vi "WS1050 16 DUT VSA-CV Sweep HD_Cycling_Ver1.4.vi"() -> ()   [LabVIEW 2012]
uses:
  WS_VCAP Driver 024/Source/WSVCAP Shell/Type Defs/WSVCAP SHL I2C DUT Mask Mode Enum.ctl
  <vilib>/Utility/file.llb/Read From Spreadsheet File (DBL).vi
  Type Def/Test Sequences.ctl
panel:
  out "VISA resource name out":refnum<visa-resource-name>="GPIB0::3::INSTR"
  out "date string":string="5/19/2014"
  out "PS1 Out":refnum<visa-resource-name>
  out "Ke2000 Out":refnum<visa-resource-name>="GPIB0::9::INSTR"
  in  "Tab Control":enum32{"Inst Control", "Data Output", "Graphs"}(tab)
  in  "Test Sequences":T1
  in  "Bank to HD":u16(ring) items=["All OFF", "All ON", "Bank_C1", "Bank_C2", "Bank_C3"]
  out "AD7747 Values":string[][](table)
  in  "Lot#":string="4NEMB"
  in  "Wafer#":string="20-EB"
  in  "File Name":string="HD_4NEMB_25_EB_65C_44V_100DC_BRD2_150916_1"
  in  "TMN DC\\CAP Data Log File Path":path=path "C:/WS1050 16 DUT Data"
  in  "SN":string[](array[string])=["1", "2", "3", "4", "5", "6", "7", "8", "9", "10", "11", "12", "13", "14", "15", "16"]
  in  "Test Program":string="WS1050 16 DUT VSA_CV Sweep HD_Cycling Ver1.4"
  out "Current Date":string="8/28/2014"
  out "Current Time":string="0950"
  in  "Start Date":string="4/24/2014"
  in  "Start Time":string="1542"
  in  "Comment":string="CV Sweep"
  in  "OK Button":bool
  in  "Calibration":bool
  in  "Control Setting":bool
  in  "CP Setting":i32(ring) items=["CP OFF", "CP ON", "CP 35V", "CP 40V", "CP 44V", "CP 50V", "DVA OFF", "DVA ON", "Reg1 ON", "Reg1 OFF", "Reg2 ON", "Reg2 OFF", "Reg3 ON", "Reg3 OFF"]
  in  "VDD(V)":dbl=3.3 format="%.3g"
  in  "Meas Clock Rate (Hz)":dbl=1000000.0 caption="Meas Speed" format="%.1p Hz"
  out "AR  Measurent(Hz)":dbl
  in  "PS1 Source":refnum<visa-resource-name>="GPIB0::5::INSTR"
  in  "Ke2000":refnum<visa-resource-name>="GPIB0::9::INSTR"
  out "Simulate FPGA":bool
  out "Online":bool
  in  "Ke2400":refnum<visa-resource-name>="GPIB0::3::INSTR"
  in  "Initialize AD7747":bool
  in  "DUT Mask Mode":T2=enum."All"
  in  "RFFE Slave Address":u8=7 caption="Slave Address" format="0x%02x"
  out "Activity Log":string="05/19/2014 -- 12:24:35.853::WSVCAP::APP::Application Started\n05/19/2014 -- 12:24:37.606::WSVCAP::WSVCAP SHL::WR I2C-REG:0x0A;MASK:0xFFFFFFFFFFFF;C1 DATA:22:22:22:22:22:22:22:22:22:22:22:22:22:22:22:22;C2 DATA:22:22:22:22:22:22:22:22:22:22:22:22:22:22:22:22;C3 DATA:22:22:22:22:22:22:22:22:22:22:22:22:22:22:22:22\r\n05/19/2014 -- 12:24:37.773::WSVCAP::WSVCAP SHL::WR I2C-ST:0,0,4,1\r\n05/19/2014 -- 12:24:37.903::WSVCAP::WSVCAP SHL::RD I2C-BYTES:4;ADD:0x00;MASK:0xFFFFFFFFFFFF\r\n05/19/2014 -- 12:24:38.045::WSVCAP::WSVCAP SHL::RD I2C:C1 DATA:2:2:2:2:2:2:2:2:2:2:2:2:2:2:2:2|A7:A9:AA:82:82:7F:82:81:82:81:83:82:81:82:82:81|46:36:BB:88:44:A3:E9:2B:32:20:ED:25:BB:3D:68:B|2C:6A:EB:A7:22:56:FE:CC:36:82:D7:B0:3B:48:F9:CC;C2 DATA:2:2:2:2:2:2:2:2:2:2:2:2:2:2:2:2|94:94:94:80:80:80:80:80:81:7E:7E:81:80:7E:80:80|47:33:15:82:62:B:E8:1C:D7:C3:7D:41:7C:B7:4C:2A|C4:B4:AE:8:1E:D1:4E:37:11:C0:6F:63:42:9D:63:B5;C3 DATA:2:2:2:2:2:2:2:2:2:2:2:2:2:2:2:2|95:95:95:81:81:7E:81:80:84:7D:80:83:81:7E:7F:80|AB:C4:14:B5:7B:52:DF:C9:79:5D:5F:30:99:31:1E:F4|6E:5C:F7:A8:C3:EB:7B:EF:33:92:89:77:4D:67:75:DD;STATUS:0:0:4:0\r\n05/19/2014 -- 12:24:38.046::WSVCAP::WSVCAP SHL::WR I2C-REG:0x0A;MASK:0xFFFFFFFFFFFF;C1 DATA:22:22:22:22:22:22:22:22:22:22:22:22:22:22:22:22;C2 DATA:22:22:22:22:22:22:22:22:22:22:22:22:22:22:22:22;C3 DATA:22:22:22:22:22:22:22:22:22:22:22:22:22:22:22:22\r\n05/19/2014 -- 12:24:38.089::WSVCAP::WSVCAP SHL::WR I2C-ST:0,0,4,1\r\n05/19/2014 -- 12:24:38.219::WSVCAP::WSVCAP SHL::RD I2C-BYTES:4;ADD:0x00;MASK:0xFFFFFFFFFFFF\r\n05/19/2014 -- 12:24:38.362::WSVCAP::WSVCAP SHL::RD I2C:C1 DATA:2:2:2:2:2:2:2:2:2:2:2:2:2:2:2:2|A7:AB:AA:82:82:82:83:83:82:82:82:82:7F:82:82:81|4B:32:96:83:3E:61:43:17:25:62:AB:4D:A2:40:2E:5|3C:76:2B:B4:EE:E4:A9:1A:AA:A:26:C7:21:2E:87:5B;C2 DATA:2:2:2:2:2:2:2:2:2:2:2:2:2:2:2:2|94:94:94:80:80:80:80:80:80:7F:80:81:80:80:7F:80|4A:32:19:7D:19:6C:79:46:61:7F:4B:B8:A5:30:F3:14|B4:70:A:8C:9C:DC:43:FA:1E:A:C6:21:A:A9:13:F3;C3 DATA:2:2:2:2:2:2:2:2:2:2:2:2:2:2:2:2|95:97:94:81:80:81:82:81:80:7E:81:84:7F:81:80:80|B2:32:D0:A7:9E:4C:AB:D4:EE:D9:F0:82:B7:91:7:FF|C1:91:B6:3D:D8:E:1B:4F:9F:6A:F1:6C:E7:3F:7:BA;STATUS:0:0:4:0\r\n05/19/2014 -- 12:24:38.364::WSVCAP::WSVCAP SHL::WR I2C-REG:0x0A;MASK:0xFFFFFFFFFFFF;C1 DATA:22:22:22:22:22:22:22:22:22:22:22:22:22:22:22:22;C2 DATA:22:22:22:22:22:22:22:22:22:22:22:22:22:22:22:22;C3 DATA:22:22:22:22:22:22:22:22:22:22:22:22:22:22:22:22\r\n05/19/2014 -- 12:24:38.406::WSVCAP::WSVCAP SHL::WR I2C-ST:0,0,4,1\r\n05/19/2014 -- 12:24:38.536::WSVCAP::WSVCAP SHL::RD I2C-BYTES:4;ADD:0x00;MASK:0xFFFFFFFFFFFF\r\n05/19/2014 -- 12:24:38.678::WSVCAP::WSVCAP SHL::RD I2C:C1 DATA:2:2:2:2:2:2:2:2:2:2:2:2:2:2:2:2|A7:A9:AB:82:82:81:82:82:82:82:82:82:82:82:82:81|46:71:4C:87:43:3D:7F:FC:25:4F:8E:54:97:3E:60:8C|AA:F4:1F:B5:CE:43:1F:36:9:87:9C:78:86:5:B6:8E;C2 DATA:2:2:2:2:2:2:2:2:2:2:2:2:2:2:2:2|94:94:94:80:7F:7F:80:80:80:80:80:81:80:80:80:80|49:36:18:7D:6E:C5:E4:3C:81:2E:41:D3:75:71:E3:72|E8:D3:E6:D1:E0:48:AE:D4:54:D:E8:8E:B4:41:68:4;C3 DATA:2:2:2:2:2:2:2:2:2:2:2:2:2:2:2:2|95:95:95:81:7F:7F:81:81:81:81:81:84:81:81:82:81|B3:F5:90:AB:82:69:7B:93:D0:77:E8:D5:E8:8C:84:E8|B9:AC:EE:2B:B6:71:8F:4A:74:31:56:BB:8A:B7:A0:C8;STATUS:0:0:4:0\r\n05/19/2014 -- 12:24:38.681::WSVCAP::WSVCAP SHL::WR I2C-REG:0x0A;MASK:0xFFFFFFFFFFFF;C1 DATA:22:22:22:22:22:22:22:22:22:22:22:22:22:22:22:22;C2 DATA:22:22:22:22:22:22:22:22:22:22:22:22:22:22:22:22;C3 DATA:22:22:22:22:22:22:22:22:22:22:22:22:22:22:22:22\r\n05/19/2014 -- 12:24:38.723::WSVCAP::WSVCAP SHL::WR I2C-ST:0,0,4,1\r\n05/19/2014 -- 12:24:38.854::WSVCAP::WSVCAP SHL::RD I2C-BYTES:4;ADD:0x00;MASK:0xFFFFFFFFFFFF\r\n05/19/2014 -- 12:24:38.996::WSVCAP::WSVCAP SHL::RD I2C:C1 DATA:2:2:2:2:2:2:2:2:2:2:2:2:2:2:2:2|A7:A9:AA:82:82:7F:83:81:82:81:84:82:7F:82:7F:82|43:FB:E:7F:3C:AD:35:35:26:A2:6C:21:4B:3D:8:6|63:9A:E1:F3:95:32:91:42:90:3C:78:1F:5C:D7:5F:D8;C2 DATA:2:2:2:2:2:2:2:2:2:2:2:2:2:2:2:2|94:94:94:80:80:80:80:80:81:80:7E:81:80:7E:7F:80|48:36:18:7F:5E:3D:69:83:DE:AE:A1:9E:31:AE:BB:96|15:A0:44:17:13:FD:CC:C8:6D:B2:EF:A7:C:C7:3B:F;C3 DATA:2:2:2:2:2:2:2:2:2:2:2:2:2:2:2:2|95:96:94:81:81:7E:82:80:84:80:80:84:7F:7E:7D:82|AD:3B:6D:A9:7C:57:9D:F5:7A:96:23:5C:36:2D:ED:5A|CD:46:DB:3B:C7:BD:70:60:33:B8:B:F7:63:A:51:4D;STATUS:0:0:4:0\r\n05/19/2014 -- 12:24:38.998::WSVCAP::WSVCAP SHL::WR I2C-REG:0x0A;MASK:0xFFFFFFFFFFFF;C1 DATA:22:22:22:22:22:22:22:22:22:22:22:22:22:22:22:22;C2 DATA:22:22:22:22:22:22:22:22:22:22:22:22:22:22:22:22;C3 DATA:22:22:22:22:22:22:22:22:22:22:22:22:22:22:22:22\r\n05/19/2014 -- 12:24:39.040::WSVCAP::WSVCAP SHL::WR I2C-ST:0,0,4,1\r\n05/19/2014 -- 12:24:39.170::WSVCAP::WSVCAP SHL::RD I2C-BYTES:4;ADD:0x00;MASK:0xFFFFFFFFFFFF\r\n05/19/2014 -- 12:24:39.311::WSVCAP::WSVCAP SHL::RD I2C:C1 DATA:2:2:2:2:2:2:2:2:2:2:2:2:2:2:2:2|A7:AA:AB:82:82:81:82:81:82:81:82:82:82:82:7F:82|44:F1:90:87:45:44:C8:2C:2C:F1:FC:1B:94:3B:3C:75|4A:49:95:19:99:73:64:3:23:24:F3:A2:5E:7F:C4:B6;C2 DATA:2:2:2:2:2:2:2:2:2:2:2:2:2:2:2:2|94:94:94:80:80:80:80:7F:80:80:7E:80:80:7E:7F:80|4C:36:17:7D:A8:9F:DE:C7:53:6D:8A:F4:41:A5:C6:E0|90:2E:24:C:D9:22:E4:76:3B:40:1D:53:33:B1:3E:4D;C3 DATA:2:2:2:2:2:2:2:2:2:2:2:2:2:2:2:2|95:97:95:81:81:7F:81:80:80:81:7F:82:81:7E:7D:82|AE:2B:A7:AB:CC:CD:A4:38:FD:17:80:F2:92:2D:45:C4|76:E5:D:B9:AD:B5:BA:8D:28:32:9E:42:B7:20:4A:D9;STATUS:0:0:4:0\r\n05/19/2014 -- 12:24:39.313::WSVCAP::WSVCAP SHL::WR I2C-REG:0x0A;MASK:0xFFFFFFFFFFFF;C1 DATA:22:22:22:22:22:22:22:22:22:22:22:22:22:22:22:22;C2 DATA:22:22:22:22:22:22:22:22:22:22:22:22:22:22:22:22;C3 DATA:22:22:22:22:22:22:22:22:22:22:22:22:22:22:22:22\r\n05/19/2014 -- 12:24:39.355::WSVCAP::WSVCAP SHL::WR I2C-ST:0,0,4,1\r\n05/19/2014 -- 12:24:39.486::WSVCAP::WSVCAP SHL::RD I2C-BYTES:4;ADD:0x00;MASK:0xFFFFFFFFFFFF\r\n05/19/2014 -- 12:24:39.628::WSVCAP::WSVCAP SHL::RD I2C:C1 DATA:2:2:2:2:2:2:2:2:2:2:2:2:2:2:2:2|A7:A9:AA:82:82:82:83:82:82:82:82:82:7F:82:7F:82|47:18:E4:87:3E:E7:6:65:25:92:37:38:A8:3E:89:85|7C:A7:7:2B:A3:7A:EC:EF:89:ED:F4:D3:D8:BC:3A:F5;C2 DATA:2:2:2:2:2:2:2:2:2:2:2:2:2:2:2:2|94:94:94:80:7F:80:80:7F:81:80:7E:80:80:80:81:80|49:37:17:80:76:25:6A:F8:DF:55:97:4D:B8:5B:2B:B1|13:E3:9A:3E:1A:2D:4F:B6:DB:E9:61:FA:8B:D6:9:CC;C3 DATA:2:2:2:2:2:2:2:2:2:2:2:2:2:2:2:2|95:95:95:81:7F:80:82:81:84:80:7F:81:80:81:7F:82|AF:93:3B:AF:5B:11:82:E4:7E:C3:2D:72:9:96:D9:A|DB:96:F2:10:5F:64:9A:C6:98:12:27:7D:10:D3:20:D9;STATUS:0:0:4:0\r\n05/19/2014 -- 12:24:40.132::WSVCAP::WSVCAP SHL::CLOSE\r\n"
  in  "C1 Cap DAC":u8=128 caption="B Data In" format="0x%02x"
  in  "C2 Cap DAC":u8=128 caption="B Data In" format="0x%02x"
  in  "C3 Cap DAC":u8=128 caption="B Data In" format="0x%02x"
  out "IDD Brd(uA)":string
  in  "VSA_IDD(A)":dbl=0.1
  in  "Stress Voltage(V)":dbl
  in  "Reset PS":bool
  in  "CP Freq":u16(ring)=3 items=["000", "001", "010", "011", "100", "101", "110", "111"]
  in  "HD/Cycling":bool
  in  "Cyc Clock Rate (Hz)":dbl=5000000.0 caption="Cycle Speed" format="%.1p Hz"
  in  "CP to HD/Cycle":i32(ring)=4 items=["CP HDC 35V", "CP HDC 40.25V", "CP HDC 27.5V", "CP HDC 30.5V", "CP HDC 44V", "CP HDC 50V"]
  in  "Bank to Cycle":u16(ring)=1 items=["Cycle All", "Cycle F12+S1", "Cycle All - F12"]
  in  "Duty Cycle %":enum16{"25", "33", "50", "75"}(ring)=enum."50"
  out "STATUS":string="Idle...."
  in  "stop":bool
  out "C1 Min_T0":string[](array[string])
  out "CAP_Value(pF)":string[][](array[string])
  out "C3 Min_T0":string[](array[string])
  out "C2 Min_T0":string[](array[string])
  in  "Abort":bool
  out "error out 2":errorcluster
  in  "Set Stress to\nComplete(Cyc/Min)":u64=8100
  out "Verify Test Condition":string[](array[string])
  out "CMin+VCAP":string[][](table)
  out "Verify Drivers to Stress":string[](array[string])
  out "Cycle Count":u64 min=1 max=4 step=1
  out "Stress \nCompleted(Min)":u64
  out "Previous Time":string="12:20:26 PM"
  out "Delta CAP_T0(pF)":dbl[][](array[numeric])
  out "Delta CAP_Tc(pF)":dbl[][](array[numeric])
  in  "error in (no error)":errorcluster
  out "error out":errorcluster
  out "CP_IDD(uA)":string
  # "Company:  WiSpry Inc 20 Fairbanks \nSte 198 Irvine CA 92618\n\nAuthor:  Andy V Tran\nCreated:  01/07/2016\nLabVIEW 2012 Pro\nTP:  WS1050 16 DUT VSA_CV Sweep HD_Cycling Ver1.3\nFPGA Version: WS_VCAP Driver 024"
  # "Note:  Ver1.0 is a original version.\n\n1.  Two look up tables, \n      a.  1st is for Stress\n      b.  2nd is for Voltage sweep\n\nVer1.1\n\n1.  No Voltage to CAP Head for initial read point\n\nVer1.2\n\n1.  Add CP Freq\n\nVer1.3\n\n1.  Add Cycling Stress\n\nSet up and Test Sequences:\n\n1.  Calibration with Empty Sockets\n2.  Load Parts\n3.  Set condition to stress (CP Voltage, Drivers to Stress, CP to stress...)\n4.  Set Date/Time to start stressing\n5.  Set TTF to stop stressing (default = 135 hrs)"
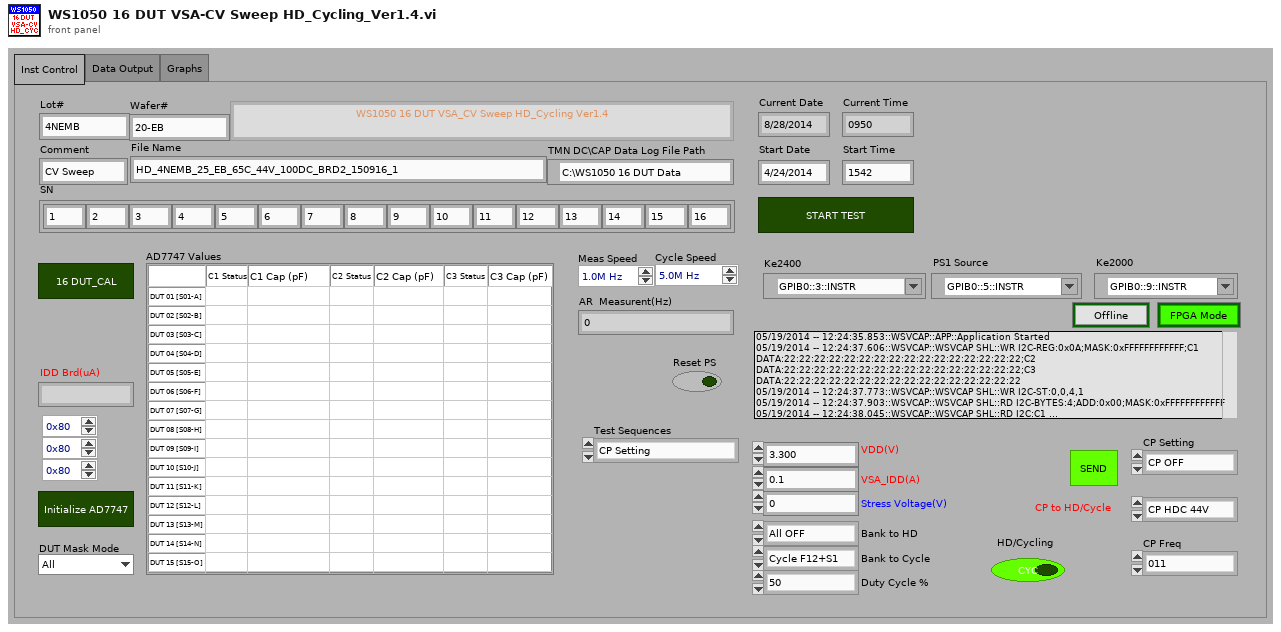
[diagram p1: front panel]
types:
  T1 = typedef "Test Sequences.ctl" = enum16{"CP Setting", "Stress", "Meas_IDD", "Meas_Cap", "Save Data", "Plot", "Idle..."}
  T2 = typedef "WSVCAP SHL I2C DUT Mask Mode Enum.ctl" = enum16{"Custom", "C1", "C2", "C3", "All"}
  T3 = typedef "WSVCAP SHL Core System Cluster.ctl" = cluster{"Settings":T4, "FPGA Resource":tag, "Online":bool, "I2C Wait Ticks":u32, "SPI Wait Ticks":u32, "RFFE Wait Ticks":u32}
  T4 = typedef "WSVCAP SHL I2C Settings Cluster.ctl" = cluster{"FPGA Resource Name":string, "I2C Slave Address":u8, "I2C Clock Rate (Hz)":dbl, "SPI Clock Rate (Hz)":dbl, "RFFE Slave Address":u8, "RFFE Clock Rate (Hz)":dbl, "Simulate FPGA":bool, "C1 Cap DAC Default":u8, "C2 Cap DAC Default":u8, "C3 Cap DAC Default":u8}
  T5 = enum16{"Idle...", "Voltage 1", "Voltage 2", "Voltage 3"}[]
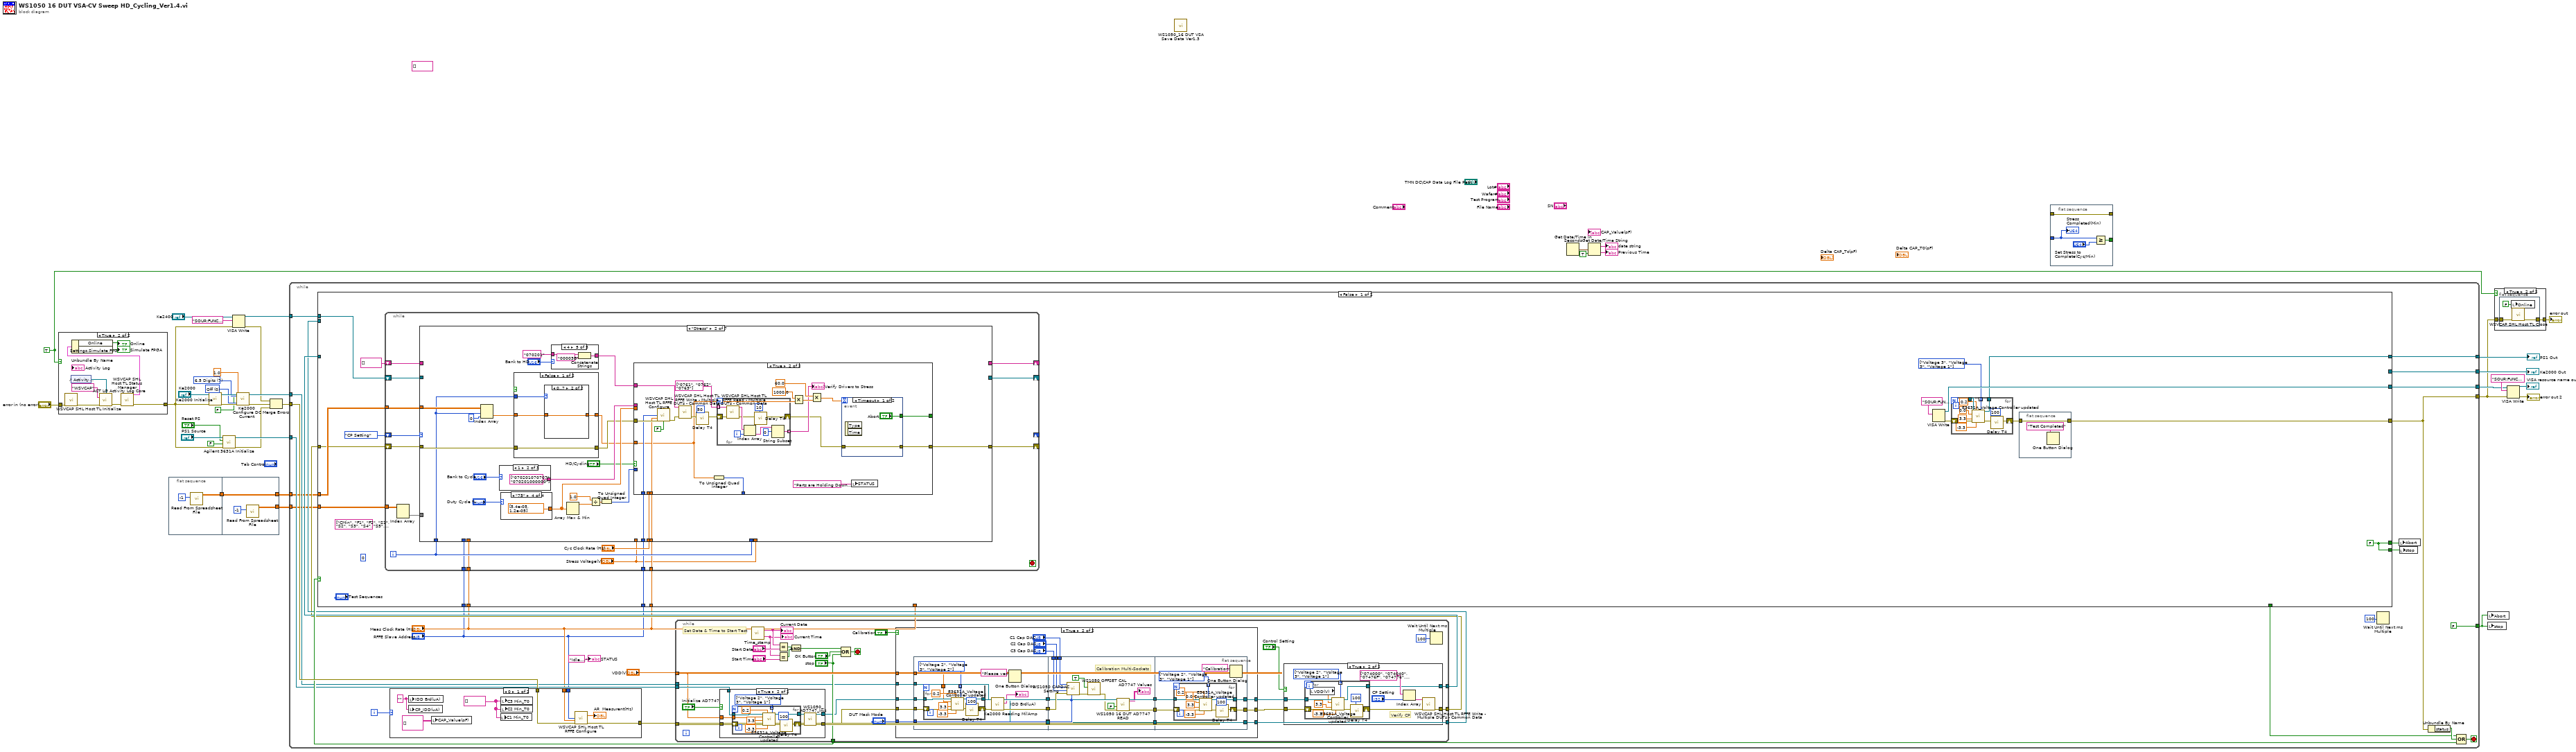
[diagram p0: block diagram]
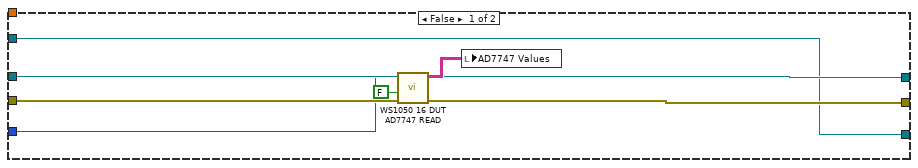
[diagram p7: hidden frame]
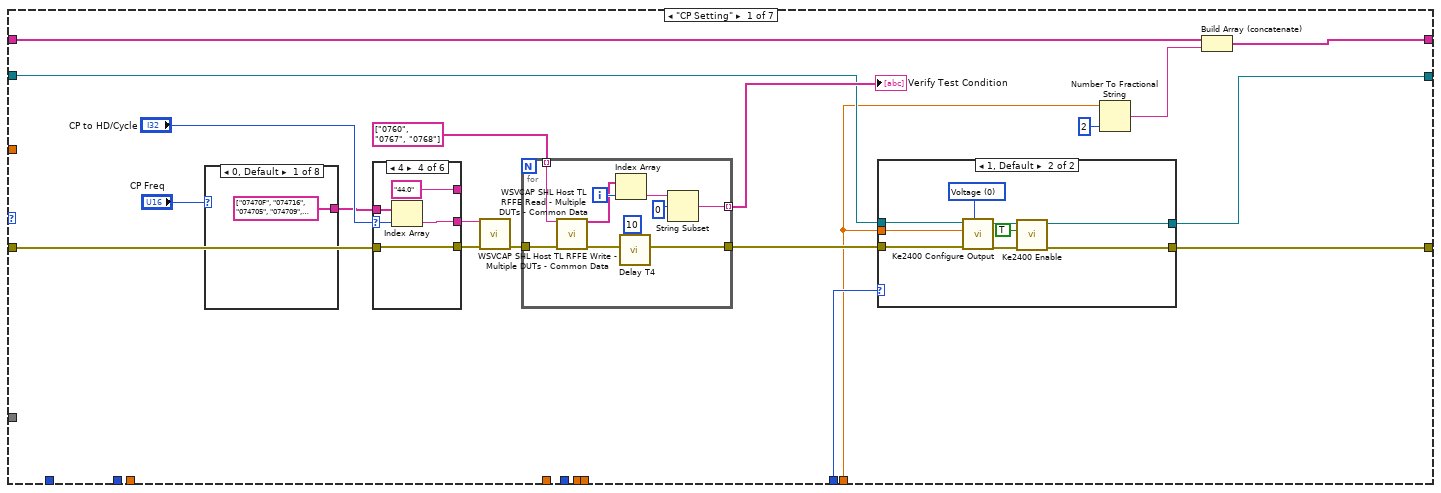
[diagram p8: hidden frame]
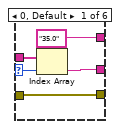
[diagram p10: hidden frame]
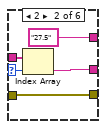
[diagram p11: hidden frame]
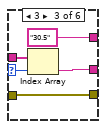
[diagram p12: hidden frame]
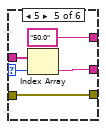
[diagram p13: hidden frame]
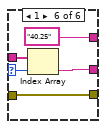
[diagram p14: hidden frame]
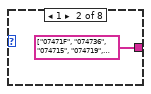
[diagram p15: hidden frame]
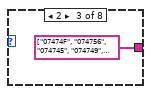
[diagram p16: hidden frame]
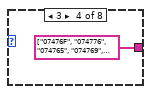
[diagram p17: hidden frame]
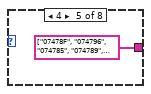
[diagram p18: hidden frame]
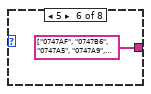
[diagram p19: hidden frame]
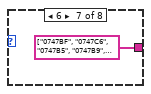
[diagram p20: hidden frame]
diagram:
  (unwired) string[] []
  w30 = TRUE
  w36 = u16 0 items=["Off", "Moving Filter", "Repeating Filter"] ("Digital Filter (0: Off)")
  w37 = u16 7 items=["3.5 Digits"=4, "4.5 Digits"=5, "5.5 Digits"=6, "6.5 Digits"=7] ("Resolution (7: 6.5 digits)")
  n1 = case shown="True" w30 {
    tunnel: "error in (no error)" -> [w44 w45]
    tunnel: [w44 w52] -> w19
    frame False {
    }
    frame True {
      n2 = call "WSVCAP SHL Host TL Initialize.vi"("error in"=w45) -> ("error out"=w46:errorcluster)  [unwired: 13 in, 1 out]
      n3 = control-ref of="Activity Log"() -> (w48:refnum<vi>)
      n4 = call "ACT LG Activity Log Core.vi"("Display Ref"=w48, "Source"="WSVCAP", "Error In (no error)"=w46) -> ("Error Out"=w47:errorcluster)  [unwired: 11 in, 1 out]
      n5 = call "WSVCAP SHL Host TL Status Manager.vi"("error in"=w47) -> ("System Out"=w53:T3, "error out"=w52:errorcluster)  [unwired: 13 in]
      n6 = Unbundle By Name(w53) -> ("Online"=→"Online":bool, "Settings.Simulate FPGA"=→"Simulate FPGA":bool)
    }
  }
  n7 = flat-sequence {
    tunnel: [w55] -> w14
    tunnel: w14 -> [w58]
    tunnel: [w58] -> w13
    tunnel: [w57] -> w12
    frame #0 {
      n8 = call-poly <vilib>:"Read From Spreadsheet File.vi"("number of rows (all:-1)"=-1) -> ("all rows"=w55:dbl[][])  [unwired: 6 in, 4 out]
    }
    frame #1 {
      n9 = call-poly <vilib>:"Read From Spreadsheet File.vi"("number of rows (all:-1)"=-1) -> ("all rows"=w57:dbl[][])  [unwired: 6 in, 4 out]
    }
  }
  n10 = call "Ke2000 Initialize.vi"("error in (no error)"=w19, "VISA resource name"="Ke2000") -> ("error out"=w38:errorcluster, "VISA resource name out"=w39:refnum<visa-resource-name>)  [unwired: 8 in]
  n11 = call "Agilent 3631A Initialize.vi"("error in (no error)"=w19, "Default"=FALSE ("Reset? (T: Yes)"), "Reset"="Reset PS", "VISA resource name"="PS1 Source") -> ("error out"=w18:errorcluster, "VISA resource name out"=w42:refnum<visa-resource-name>)  [unwired: 6 in]
  n12 = VISA Write(VISA resource name="Ke2400", write buffer="SOUR:FUNC VOLT;VOLT:MODE FIX;RANG 100;LEV 0.0;:SENS:FUNC \"CURR\";CURR:PROT 60E-3;RANG 100E-3;:OUTP ON", error in (no error)=w19) -> (VISA resource name out=w27:refnum<visa-resource-name>, error out=w22:errorcluster)  [unwired: 1 out]
  n13 = call "Ke2000 Configure DC Current.vi"("Resolution (7: 6.5 digits)"=w37, "Digital Filter (0: Off)"=w36, "Auto Range? (T: Auto)"=FALSE, "error in"=w38, "Custom Range (0 A)"=1.0, "VISA resource name"=w39) -> ("error out"=w20:errorcluster, "VISA resource name out"=w34:refnum<visa-resource-name>)  [unwired: 4 in]
  n14 = Merge Errors(w22, w20, w18) -> (w28:errorcluster)
  n15 = while {
    tunnel: w28 -> [w79]
    tunnel: [w69] -> w24
    tunnel: w42 -> [w73]
    tunnel: w34 -> [w74]
    tunnel: [w82] -> w33
    tunnel: [w81] -> w32
    tunnel: w27 -> [w78]
    tunnel: [w77] -> w25
    tunnel: [FALSE] -> w17
    tunnel: w13 -> [w65]
    tunnel: w12 -> [w64]
    i -> [w80]
    stop <- w83 stop-if-true
    n16 = case shown="0" w80 {
      tunnel: w79 -> [w93 w94]
      tunnel: [w92 w94] -> w75
      tunnel: "RFFE Slave Address" -> [w90 _]
      tunnel: "Meas Clock Rate (Hz)" -> [w86 _]
      frame 0 {
        w89 = string[] []
        w87 = "" ("uA")
        n17 = local write "IDD Brd(uA)"(w87) -> ()
        n18 = local write "CP_IDD(uA)"(w87) -> ()
        n19 = local write "CAP_Value(pF)"(string[][] []) -> ()
        n20 = local write "C1 Min_T0"(w89) -> ()
        n21 = local write "C3 Min_T0"(w89) -> ()
        n22 = local write "C2 Min_T0"(w89) -> ()
        n23 = call "WSVCAP SHL Host TL RFFE Configure.vi"("RFFE Slave Address"=w90, "Clock Rate (Hz)"=w86, "error in"=w93) -> ("Actual Rate (Hz)"=→"AR  Measurent(Hz)":dbl, "error out"=w92:errorcluster)  [unwired: 11 in]
      }
      frame 1, Default {
      }
    }
    n24 = while {
      tunnel: ["stop"] -> w76
      tunnel: w75 -> [w106]
      tunnel: [w98] -> w70
      tunnel: w73 -> [w104]
      tunnel: w74 -> [w100]
      tunnel: [w101] -> w72
      tunnel: [w99] -> w71
      tunnel: "VDD(V)" -> [w96]
      stop <- w113 stop-if-true
      # "Set Date & Time to Start Test"
      n25 = case shown="True" "Initialize AD7747" {
        tunnel: w106 -> [w122 w128]
        tunnel: [w122 w124] -> w105
        tunnel: w104 -> [w121 w126]
        tunnel: [w121 w125] -> w103
        tunnel: w96 -> [_ w123]
        frame False {
        }
        frame True {
          w129 = T5 [enum."Voltage 2", enum."Voltage 3", enum."Voltage 1"] items=["Idle...", "Voltage 1", "Voltage 2", "Voltage 3"]
          n26 = for {
            tunnel: w126 -> [w139]
            tunnel: w129 -> [w137] mode=indexing
            tunnel: [w136] -> w125
            shift-right: [w133] -> w127
            shift-left: w128 -> [w140]
            tunnel: w123 -> [w131]
            n27 = call "E3631A_Voltage Controller updated.vi"("VISA resource name"=w139, "I_VDD(A)"=0.2, "Channel Controller"=w137, "Voltage 1"=w131, "Voltage 2"=3.3, "error in (no error)"=w140, "Voltage 3"=-3.3) -> ("VISA resource name out"=w136:refnum<visa-resource-name>, "error out"=w132:errorcluster)  [unwired: 7 in]
            n28 = call "Delay T4.vi"("milliseconds to wait"=u32 100, "error in (no error)"=w132) -> ("error out"=w133:errorcluster)  [unwired: 9 in]
          }
          n29 = call "WS1050_AD7747_Init.vi"("error in"=w127) -> ("error out"=w124:errorcluster)  [unwired: 10 in]
        }
      }
      n30 = call "Time_stamp.vi"() -> ("date/time string"=w118:string, "date string"=w120:string)  [unwired: 2 in]
      "Current Date" <- w120
      "Current Time" <- w118
      n31 = Equal?(x=w120, y="Start Date") -> (x = y?=w116:bool)
      n32 = Equal?(x=w118, y="Start Time") -> (x = y?=w115:bool)
      n33 = And(x=w116, y=w115) -> (x .and. y?=w112:bool)
      n34 = Compound Arithmetic op=OR(w112, "OK Button", "stop") -> (w113:bool)
      n35 = case shown="True" "Calibration" {
        tunnel: w105 -> [w167 w186]
        tunnel: [w166 w183] -> w97
        tunnel: w103 -> [w165 w182]
        tunnel: "DUT Mask Mode" -> [w164 w178]
        tunnel: [w165 w177] -> w102
        tunnel: w100 -> [w163 w173]
        tunnel: [w163 w170] -> w99
        tunnel: w96 -> [_ w169]
        frame False {
          n36 = call "WS1050 16 DUT AD7747 READ.vi"("error in"=w167, "Log (T)"=FALSE, "DUT Mask Mode (All)"=w164) -> ("error out"=w166:errorcluster, "AD7747 Values"=w168:string[][])  [unwired: 7 in]
          n37 = local write "AD7747 Values"(w168) -> ()
        }
        frame True {
          n38 = flat-sequence {
            tunnel: w186 -> [w196]
            tunnel: [w191] -> w185
            tunnel: w182 -> [w195]
            tunnel: [w194] -> w181
            tunnel: w178 -> [w193]
            tunnel: [w193] -> w179
            tunnel: w173 -> [w189]
            tunnel: [w188] -> w172
            tunnel: w169 -> [w187]
            tunnel: w185 -> [w222]
            tunnel: [w221] -> w184
            tunnel: w181 -> [w220]
            tunnel: [w220] -> w180
            tunnel: w179 -> [w219]
            tunnel: "C1 Cap DAC" -> [w215]
            tunnel: "C2 Cap DAC" -> [w214]
            tunnel: "C3 Cap DAC" -> [w213]
            tunnel: w172 -> [w212]
            tunnel: [w212] -> w171
            tunnel: w184 -> [w225]
            tunnel: [w228] -> w183
            tunnel: w180 -> [w227]
            tunnel: [w224] -> w177
            tunnel: w171 -> [w223]
            tunnel: [w223] -> w170
            frame #0 {
              w197 = T5 [enum."Voltage 2", enum."Voltage 3", enum."Voltage 2"] items=["Idle...", "Voltage 1", "Voltage 2", "Voltage 3"]
              n39 = for {
                tunnel: w195 -> [w208]
                tunnel: w197 -> [w205] mode=indexing
                tunnel: [w204] -> w194
                shift-right: [w202] -> w190
                shift-left: w196 -> [w209]
                tunnel: w187 -> [w199]
                n40 = call "E3631A_Voltage Controller updated.vi"("VISA resource name"=w208, "I_VDD(A)"=0.2, "Channel Controller"=w205, "Voltage 1"=w199, "Voltage 2"=3.3, "error in (no error)"=w209, "Voltage 3"=-3.3) -> ("VISA resource name out"=w204:refnum<visa-resource-name>, "error out"=w201:errorcluster)  [unwired: 7 in]
                n41 = call "Delay T4.vi"("milliseconds to wait"=u32 100, "error in (no error)"=w201) -> ("error out"=w202:errorcluster)  [unwired: 9 in]
              }
              n42 = call "Ke2000 Reading MilAmp.vi"("error in (no error)"=w190, "VISA resource name"=w189) -> ("error out"=w191:errorcluster, "uA"=→"IDD Brd(uA)":string, "VISA resource name out"=w188:refnum<visa-resource-name>)  [unwired: 7 in]
              n43 = One Button Dialog(message="Please verify all sockets should be empty...") -> ()  [unwired: 1 in, 1 out]
            }
            frame #1 {
              # "Calibration Multi-Sockets"
              n44 = call "WS1050 CAPDAC Setting.vi"("DUT Mask Mode (All)"=w219, "error in"=w222, "C3 Cap DAC"=w213, "C2 Cap DAC"=w214, "C1 Cap DAC"=w215) -> ("error out"=w217:errorcluster)  [unwired: 5 in, 1 out]
              n45 = call "WS1050 OFFSET CAL.vi"("error in"=w217, "OFFSET CAL"=TRUE ("Read?")) -> ("error out"=w216:errorcluster)  [unwired: 8 in, 1 out]
              n46 = call "WS1050 16 DUT AD7747 READ.vi"("error in"=w216, "Log (T)"=FALSE, "DUT Mask Mode (All)"=w219) -> ("error out"=w221:errorcluster, "AD7747 Values"=→"AD7747 Values":string[][])  [unwired: 7 in]
            }
            frame #2 {
              w226 = T5 [enum."Voltage 2", enum."Voltage 3", enum."Voltage 1"] items=["Idle...", "Voltage 1", "Voltage 2", "Voltage 3"]
              n47 = for {
                tunnel: w227 -> [w240]
                tunnel: w226 -> [w236] mode=indexing
                tunnel: [w235] -> w224
                shift-right: [w231] -> w228
                shift-left: w225 -> [w237]
                n48 = call "E3631A_Voltage Controller updated.vi"("VISA resource name"=w240, "I_VDD(A)"=0.2, "Channel Controller"=w236, "Voltage 1"=0.0, "Voltage 2"=3.3, "error in (no error)"=w237, "Voltage 3"=-3.3) -> ("VISA resource name out"=w235:refnum<visa-resource-name>, "error out"=w230:errorcluster)  [unwired: 7 in]
                n49 = call "Delay T4.vi"("milliseconds to wait"=u32 100, "error in (no error)"=w230) -> ("error out"=w231:errorcluster)  [unwired: 9 in]
              }
              n50 = One Button Dialog(message="Calibration Completed....") -> ()  [unwired: 1 in, 1 out]
            }
          }
        }
      }
      n51 = case shown="True" "Control Setting" {
        tunnel: [w141 w144] -> w98
        tunnel: w102 -> [w142 w147]
        tunnel: [w142 w145] -> w101
        tunnel: w97 -> [w141 w143]
        frame False {
        }
        frame True {
          w148 = T5 [enum."Voltage 2", enum."Voltage 3", enum."Voltage 1"] items=["Idle...", "Voltage 1", "Voltage 2", "Voltage 3"]
          # "Verify CP"
          n52 = for {
            tunnel: w147 -> [w160]
            tunnel: w148 -> [w157] mode=indexing
            shift-right: [w154] -> w146
            shift-left: w143 -> [w161]
            tunnel: [w152] -> w145
            n53 = local read "VDD(V)"() -> (w156:dbl)
            n54 = call "E3631A_Voltage Controller updated.vi"("VISA resource name"=w160, "Channel Controller"=w157, "Voltage 1"=w156, "Voltage 2"=3.3, "error in (no error)"=w161, "Voltage 3"=-3.3) -> ("VISA resource name out"=w152:refnum<visa-resource-name>, "error out"=w155:errorcluster)  [unwired: 8 in]
            n55 = call "Delay T4.vi"("milliseconds to wait"=u32 100, "error in (no error)"=w155) -> ("error out"=w154:errorcluster)  [unwired: 9 in]
          }
          n56 = Index Array(array=string[] ["074000", "074040", "07476F", "074776", "07477B", "07477C", "074820", "074800", "07413B", "074100", "07423B", "074200", "07433B", "074300"], index="CP Setting") -> (element=w149:string)
          n57 = call "WSVCAP SHL Host TL RFFE Write - Multiple DUTs - Common Data.vi"("Data Out"=w149, "error in"=w146) -> ("error out"=w144:errorcluster)  [unwired: 13 in]
        }
      }
      n58 = Wait Until Next ms Multiple(millisecond multiple=u32 100) -> ()  [unwired: 1 out]
    }
    n59 = case shown="False" w76 {
      tunnel: w70 -> [w242 w640]
      tunnel: [w251 w640] -> w69
      tunnel: w72 -> [_ w638]
      tunnel: w71 -> [_ w639]
      tunnel: [_ w639] -> w82
      tunnel: [w253 w638] -> w81
      tunnel: w78 -> [w243 w637]
      tunnel: [w257 w637] -> w77
      tunnel: [w256 w636] -> w67
      tunnel: [w256 w636] -> w66
      tunnel: w65 -> [w249 _]
      tunnel: w64 -> [w248 _]
      tunnel: [_ w636] -> w62
      tunnel: "RFFE Slave Address" -> [w247 _]
      tunnel: "Meas Clock Rate (Hz)" -> [_ _]
      tunnel: "Meas Clock Rate (Hz)" -> [w246 _]
      tunnel: "Meas Clock Rate (Hz)" -> [w245 _]
      tunnel: "RFFE Slave Address" -> [w244 _]
      frame False {
        (unwired) string[] ["CMin", "F1", "F2", "S1", "S2", "S3", "S4", "S5", "S6", "S7", "S8", "S9", "S10", "S11", "S12", "S13", "S14", "S14F12", "All OFF"]
        w255 = T5 [enum."Voltage 3", enum."Voltage 3", enum."Voltage 1"] items=["Idle...", "Voltage 1", "Voltage 2", "Voltage 3"]
        (unwired) u64 0 ("disabled index (col)")
        w256 = FALSE
        n60 = while {
          shift-right: _ -> [_]
          shift-left: Test_Sequences."CP Setting" ("Test Sequences") -> [w275]
          shift-right: [w274] -> _
          shift-left: string[] [] -> [w273]
          shift-right: [w272] -> _
          shift-left: w242 -> [w271]
          shift-right: [w270] -> _
          shift-left: w243 -> [w269]
          tunnel: w249 -> [w266]
          tunnel: w248 -> [w260]
          tunnel: w247 -> [w265]
          tunnel: w246 -> [w264]
          tunnel: w245 -> [w263]
          tunnel: w244 -> [w262]
          i -> [w267]
          stop <- _ stop-if-true
          n61 = Index Array(array=w260) -> (element=w259:dbl[])  [unwired: 2 in]
          n62 = case shown="\"Stress\"" w275 {
            tunnel: w273 -> [w283 _ _ _ _ _ _]
            tunnel: [w282 _ _ _ _ _ _] -> w274
            tunnel: [w281 w360 w492 _ _ _ _] -> w272
            tunnel: w271 -> [w280 w370 w500 _ _ _ _]
            tunnel: w269 -> [w279 _ w499 _ _ _ _]
            tunnel: [w278 _ w493 _ _ _ _] -> w270
            tunnel: w267 -> [w277 _ _ _ _ _ _]
            tunnel: "Cyc Clock Rate (Hz)" -> [_ w369 _ _ _ _ _]
            tunnel: w267 -> [_ w355 w498 _ _ _ _]
            tunnel: w266 -> [_ w359 _ _ _ _ _]
            tunnel: w265 -> [_ w358 _ _ _ _ _]
            tunnel: w264 -> [_ w357 _ _ _ _ _]
            tunnel: w263 -> [_ _ w496 _ _ _ _]
            tunnel: w262 -> [_ _ w495 _ _ _ _]
            tunnel: "Stress Voltage(V)" -> [w276 _ _ _ _ _ _]
            tunnel: "Stress Voltage(V)" -> [_ _ _ _ _ _ _]
            tunnel: w259 -> [_ _ w491 _ _ _ _]
            frame "CP Setting" {
              n63 = case shown="0, Default" "CP Freq" {
                tunnel: [string[] ["07470F", "074716", "074705", "074709", "07471B", "07471C"] string[] ["07471F", "074736", "074715", "074719", "07473B", "07473C"] string[] ["07474F", "074756", "074745", "074749", "07475B", "07475C"] string[] ["07476F", "074776", "074765", "074769", "07477B", "07477C"] string[] ["07478F", "074796", "074785", "074789", "07479B", "07479C"] string[] ["0747AF", "0747B6", "0747A5", "0747A9", "0747BB", "0747BC"] string[] ["0747BF", "0747C6", "0747B5", "0747B9", "0747CB", "0747CC"] string[] ["0747EF", "0747F6", "0747E5", "0747E9", "0747FB", "0747FC"]] -> w292
                frame 0, Default {
                }
                frame 1 {
                }
                frame 2 {
                }
                frame 3 {
                }
                frame 4 {
                }
                frame 5 {
                }
                frame 6 {
                }
                frame 7 {
                }
              }
              n64 = case shown="4" "CP to HD/Cycle" {
                selector: "CP to HD/Cycle" -> [w319 w324 w329 w334 w339 w343]
                tunnel: w292 -> [w320 w325 w330 w335 w340 w345]
                tunnel: [w318 w323 w328 w333 w338 w344] -> w290
                tunnel: ["35.0" ("Data Out") "27.5" ("Data Out") "30.5" ("Data Out") "44.0" ("Data Out") "50.0" ("Data Out") "40.25" ("Data Out")] -> _
                tunnel: [w316 w321 w326 w331 w336 w341] -> w287
                tunnel: w280 -> [w316 w321 w326 w331 w336 w341]
                frame 0, Default {
                  n65 = Index Array(array=w320, index=w319) -> (element=w318:string)
                }
                frame 2 {
                  n66 = Index Array(array=w325, index=w324) -> (element=w323:string)
                }
                frame 3 {
                  n67 = Index Array(array=w330, index=w329) -> (element=w328:string)
                }
                frame 4 {
                  n68 = Index Array(array=w335, index=w334) -> (element=w333:string)
                }
                frame 5 {
                  n69 = Index Array(array=w340, index=w339) -> (element=w338:string)
                }
                frame 1 {
                  n70 = Index Array(array=w345, index=w343) -> (element=w344:string)
                }
              }
              n71 = call "WSVCAP SHL Host TL RFFE Write - Multiple DUTs - Common Data.vi"("Data Out"=w290, "error in"=w287) -> ("error out"=w291:errorcluster)  [unwired: 13 in]
              n72 = for {
                tunnel: string[] ["0760", "0767", "0768"] -> [w315] mode=indexing
                tunnel: [w311] -> w289 mode=indexing
                tunnel: w291 -> [w309]
                tunnel: [w307] -> w286
                i -> [w314]
                n73 = call "WSVCAP SHL Host TL RFFE Read - Multiple DUTs - Common Data.vi"("Data Out"=w315, "error in"=w309) -> ("RFFE Data In"=w313:string[], "error out"=w306:errorcluster)  [unwired: 12 in]
                n74 = Index Array(array=w313, index=w314) -> (element=w310:string)
                n75 = call "Delay T4.vi"("milliseconds to wait"=u32 10, "error in (no error)"=w306) -> ("error out"=w307:errorcluster)  [unwired: 9 in]
                n76 = String Subset(string=w310, offset (0)=0) -> (substring=w311:string)  [unwired: 1 in]
              }
              "Verify Test Condition" <- w289
              n77 = case shown="1, Default" w277 {
                tunnel: [w295 w302] -> w281
                tunnel: w286 -> [w295 w301]
                tunnel: w279 -> [w296 w300]
                tunnel: [w296 w299] -> w278
                tunnel: w276 -> [_ w297]
                frame 0 {
                }
                frame 1, Default {
                  w298 = u16 0 items=["Voltage", "Current"] ("Source Mode  (0: Voltage)")
                  n78 = call "Ke2400 Configure Output.vi"("Source Mode  (0: Voltage)"=w298, "error in (no error)"=w301, "Output Level (0)"=w297, "VISA resource name"=w300) -> ("error out"=w305:errorcluster, "VISA resource name out"=w303:refnum<visa-resource-name>)  [unwired: 6 in]
                  n79 = call "Ke2400 Enable.vi"("error in (no error)"=w305, "ON/OFF"=TRUE ("Enable Output (T: Enable)"), "VISA resource name"=w303) -> ("error out"=w302:errorcluster, "VISA resource name out"=w299:refnum<visa-resource-name>)  [unwired: 7 in]
                }
              }
              n80 = Number To Fractional String(number=w276, precision (6)=i16 2) -> (F-format string=w284:string)  [unwired: 2 in]
              n81 = Build Array (concatenate)(w283, w284) -> (w282:string[])
            }
            frame "Stress" {
              n82 = Index Array(array=w359, index (row)=w355, index (col)=0 ("disabled index (col)")) -> (element=w372:dbl)
              n83 = case shown="1" "Bank to Cycle" {
                tunnel: [string[] ["0702013B3B3B", "070201000000"] ("Command 2") string[] ["070201070707", "070201000000"] ("Command 2") string[] ["070201383838", "070201000000"] ("Command 2")] -> w365
                frame 0, Default {
                }
                frame 1 {
                }
                frame 2 {
                }
              }
              n84 = case shown="\"75\"" "Duty Cycle %" {
                tunnel: [dbl[] [1.2e-05, 5.4e-05] ("Set Delay 2") dbl[] [1.9e-05, 4.7e-05] ("Set Delay 2") dbl[] [3.3e-05, 3.3e-05] ("Set Delay 2") dbl[] [5.4e-05, 1.2e-05] ("Set Delay 2")] -> w364
                frame "25", Default {
                }
                frame "33" {
                }
                frame "50" {
                }
                frame "75" {
                }
              }
              n85 = case shown="False" {
                selector: _ -> [_ _]
                tunnel: w372 -> [w474 w481]
                tunnel: [w475 w480] -> w356
                tunnel: w355 -> [w473 w479]
                tunnel: w370 -> [w472 w478]
                tunnel: [w472 w478] -> w363
                frame False {
                  n86 = case shown="0..7" w473 {
                    tunnel: w474 -> [_ w477]
                    tunnel: [10000.0 w477] -> w475
                    frame 8, Default {
                    }
                    frame 0..7 {
                    }
                  }
                }
                frame True {
                  n87 = case shown="15, Default" w479 {
                    tunnel: w481 -> [_ w483]
                    tunnel: [60.0 w483] -> w480
                    frame 15, Default {
                    }
                    frame 0..14 {
                    }
                  }
                }
              }
              n88 = case shown="4" "Bank to HD" {
                tunnel: "070201" -> [w379 w381 w384 w387 w390]
                tunnel: [w377 w380 w383 w386 w389] -> w366
                frame 0, Default {
                  n89 = Concatenate Strings(w379, "000000" ("string")) -> (w377:string)
                }
                frame 1 {
                  n90 = Concatenate Strings(w381, "3B3B3B" ("string")) -> (w380:string)
                }
                frame 2 {
                  n91 = Concatenate Strings(w384, "3B0000" ("string")) -> (w383:string)
                }
                frame 3 {
                  n92 = Concatenate Strings(w387, "003B00" ("string")) -> (w386:string)
                }
                frame 4 {
                  n93 = Concatenate Strings(w390, "00003B" ("string")) -> (w389:string)
                }
              }
              n94 = Array Max & Min(array=w364) -> (max value=w373:dbl)  [unwired: 3 out]
              n95 = Divide(x=1.0, y=w373) -> (x/y=w374:dbl)
              n96 = To Unsigned Quad Integer(1:w374) -> (0:w361:u64)
              n97 = case shown="True" "HD/Cycling" {
                tunnel: [w400 w457] -> _
                tunnel: w366 -> [_ w456]
                tunnel: [w401 w455] -> w360
                tunnel: w363 -> [w397 w442]
                tunnel: w365 -> [w404 _]
                tunnel: w364 -> [w403 _]
                tunnel: w361 -> [w402 _]
                tunnel: [w399 w444] -> _
                tunnel: w369 -> [w395 _]
                tunnel: w358 -> [w394 w439]
                tunnel: w357 -> [_ w438]
                tunnel: w356 -> [w392 w437]
                frame False {
                  n98 = call "WSVCAP SHL Host TL RFFE Configure.vi"("RFFE Slave Address"=w394, "Clock Rate (Hz)"=w395, "error in"=w397, "Log (T)"=FALSE) -> ("error out"=w396:errorcluster)  [unwired: 10 in, 1 out]
                  n99 = while {
                    tunnel: w392 -> [w424]
                    tunnel: [w414] -> w401
                    tunnel: [w409] -> w400
                    tunnel: w396 -> [w422]
                    tunnel: [w413] -> w399
                    tunnel: w404 -> [w421]
                    tunnel: w403 -> [w420]
                    tunnel: w402 -> [w411]
                    i -> [w419]
                    stop <- w417 stop-if-true
                    # "Target Cycles"
                    n100 = To Unsigned Quad Integer(1:w424) -> (0:w423:u64)
                    n101 = case shown="0" w419 {
                      tunnel: [w430 w431] -> w407
                      tunnel: w422 -> [w429 w431]
                      tunnel: w421 -> [w428 _]
                      tunnel: w420 -> [w427 _]
                      frame 0 {
                        n102 = call "WSVCAP SHL Host TL RFFE Write Cycle - Multiple DUTs - Common Data1.vi"("Data Out (Cycle Commands)"=w428, "Post Command Delay"=w427, "error in"=w429) -> ("error out"=w430:errorcluster)  [unwired: 12 in]
                      }
                      frame 1, Default {
                      }
                    }
                    n103 = Multiply(x=w423, y=u64 1000) -> (x*y=w413:u64)
                    n104 = call "WSVCAP SHL Host TL SPI_RFFE Query Cycle Count.vi"("error in"=w407) -> ("Cycle Count"=w406:u64, "error out"=w405:errorcluster)  [unwired: 13 in]
                    "Cycle Count" <- w406
                    n105 = Subtract(x=w413, y=w406) -> (x-y=w412:u64)
                    n106 = Greater Or Equal?(x=w406, y=w413) -> (x >= y?=w418:bool)
                    n107 = Greater?(x=w412, y=w411) -> (0:w410:bool)
                    n108 = case shown="True" w418 {
                      tunnel: [w433 w435] -> w415
                      tunnel: w405 -> [w433 w434]
                      tunnel: [FALSE TRUE] -> w416
                      frame False {
                      }
                      frame True {
                        n109 = call "WSVCAP SHL Host TL RFFE Stop Write Cycle.vi"("error in"=w434) -> ("error out"=w435:errorcluster)  [unwired: 14 in]
                      }
                    }
                    n110 = local read "Abort"() -> (w409:bool)
                    n111 = Or(x=w416, y=w409) -> (x .or. y?=w417:bool)
                    n112 = case shown="True" w410 {
                      tunnel: w415 -> [w425 w426]
                      tunnel: [w425 w426] -> w414
                      frame False {
                      }
                      frame True {
                      }
                    }
                  }
                  n113 = local write "STATUS"("Parts are cycling...." ("STATUS")) -> ()
                }
                frame True {
                  n114 = call "WSVCAP SHL Host TL RFFE Configure.vi"("RFFE Slave Address"=w439, "Clock Rate (Hz)"=w438, "error in"=w442, "Log (T)"=FALSE) -> ("error out"=w441:errorcluster)  [unwired: 10 in, 1 out]
                  n115 = call "WSVCAP SHL Host TL RFFE Write - Multiple DUTs - Common Data.vi"("Data Out"=w456, "error in"=w441) -> ("error out"=w450:errorcluster)  [unwired: 13 in]
                  n116 = call "Delay T4.vi"("milliseconds to wait"=u32 50, "error in (no error)"=w450) -> ("error out"=w447:errorcluster)  [unwired: 9 in]
                  n117 = To Unsigned Quad Integer(1:w437) -> (0:w444:u64)
                  n118 = for {
                    tunnel: string[] ["0761", "0762", "0763"] -> [w467] mode=indexing
                    tunnel: [w463] -> w446 mode=indexing
                    shift-right: [w460] -> w445
                    shift-left: w447 -> [w466]
                    i -> [w465]
                    n119 = call "WSVCAP SHL Host TL RFFE Read - Multiple DUTs - Common Data.vi"("Data Out"=w467, "error in"=w466) -> ("RFFE Data In"=w462:string[], "error out"=w459:errorcluster)  [unwired: 12 in]
                    n120 = Index Array(array=w462, index=w465) -> (element=w461:string)
                    n121 = call "Delay T4.vi"("milliseconds to wait"=u32 10, "error in (no error)"=w459) -> ("error out"=w460:errorcluster)  [unwired: 9 in]
                    n122 = String Subset(string=w461, offset (0)=0) -> (substring=w463:string)  [unwired: 1 in]
                  }
                  "Verify Drivers to Stress" <- w446
                  n123 = Multiply(x=1000.0, y=w437) -> (x*y=w453:dbl)
                  n124 = Multiply(x=60.0, y=w453) -> (x*y=w454:dbl)
                  n125 = event shown="[0] Timeout" {
                    selector: _ -> [_ _]
                    dyn-events: _ -> [_ _]
                    timeout: w454 -> [_ _]
                    tunnel: ["Abort" TRUE ("Abort")] -> w457
                    tunnel: w445 -> [w468 w470]
                    tunnel: [w468 w470] -> w455
                    event Timeout {
                      n126 = event-data() -> ()  [unwired: 1 in, 2 out]
                    }
                    event "Abort": Value Change {
                      n127 = event-data() -> ()  [unwired: 1 in, 3 out]
                    }
                  }
                  n128 = local write "STATUS"("Parts are Holding Down...." ("STATUS")) -> ()
                }
              }
            }
            frame "Meas_IDD" {
              n129 = stacked-sequence {
                seq-local: [_ w557 _] -> [_ _ w563]
                seq-local: [w539 _ _] -> [_ w558 _]
                seq-local: [w538 _ _] -> [_ w556 _]
                seq-local: [_ w556 _] -> [_ _ w562]
                tunnel: [_ _ w579] -> w497
                tunnel: [_ _ w578] -> _
                tunnel: w500 -> [w542 _ _]
                tunnel: w495 -> [_ w561 _]
                tunnel: w496 -> [_ w560 _]
                tunnel: w498 -> [w541 _ _]
                tunnel: w499 -> [w540 _ _]
                tunnel: [_ _ w562] -> w494
                frame #0 {
                  n130 = case shown="0" w541 {
                    tunnel: [w545 w555] -> w539
                    tunnel: w542 -> [w552 w555]
                    tunnel: [w551 w554] -> w538
                    tunnel: w540 -> [w550 w554]
                    frame 0 {
                      w548 = u16 0 items=["Voltage", "Current"] ("Source Mode  (0: Voltage)")
                      n131 = call "Ke2400 Configure Output.vi"("Source Mode  (0: Voltage)"=w548, "error in (no error)"=w552, "Output Level (0)"=0.0, "VISA resource name"=w550) -> ("error out"=w553:errorcluster, "VISA resource name out"=w546:refnum<visa-resource-name>)  [unwired: 6 in]
                      n132 = call "Ke2400 Enable.vi"("error in (no error)"=w553, "ON/OFF"=TRUE ("Enable Output (T: Enable)"), "VISA resource name"=w546) -> ("error out"=w544:errorcluster, "VISA resource name out"=w551:refnum<visa-resource-name>)  [unwired: 7 in]
                      n133 = call "Delay T4.vi"("milliseconds to wait"=u32 50, "error in (no error)"=w544) -> ("error out"=w545:errorcluster)  [unwired: 9 in]
                    }
                    frame 1, Default {
                    }
                  }
                }
                frame #1 {
                  n134 = call "WSVCAP SHL Host TL RFFE Configure.vi"("RFFE Slave Address"=w561, "Clock Rate (Hz)"=w560, "error in"=w558, "Log (T)"=FALSE) -> ("error out"=w557:errorcluster)  [unwired: 10 in, 1 out]
                }
                frame #2 {
                  w574 = string[] [] ("CP Current(uA)")
                  n135 = call "WSVCAP SHL Host TL RFFE Write - Multiple DUTs - Common Data.vi"("Data Out"="070201000000", "error in"=w563) -> ("error out"=w570:errorcluster)  [unwired: 13 in]
                  n136 = call "Delay T4.vi"("milliseconds to wait"=u32 100, "error in (no error)"=w570) -> ("error out"=w571:errorcluster)  [unwired: 9 in]
                  n137 = local write "CP_IDD(uA)"("" ("CP_IDD(uA)")) -> ()
                  n138 = for {
                    tunnel: string[] ["00", "01", "02", "04", "08", "0C", "10", "14", "18", "1C", "20", "24", "28", "2C", "30", "34", "38", "3B", "00"] -> [w582] mode=indexing
                    tunnel: [w581] -> w578 mode=indexing
                    shift-right: [w580] -> w575
                    shift-left: w571 -> [w580]
                    n139 = Concatenate Strings("070201" ("string"), w582, w582, w582) -> (w581:string)
                  }
                  n140 = local write "CAP_Value(pF)"(string[][] [] ("VSA_Value(pF)")) -> ()
                  n141 = call "WS1050 16 DUT AD7747 READ.vi"("error in"=w575, "Log (T)"=FALSE, "DUT Mask Mode (All)"=WSVCAP_SHL_I2C_DUT_Mask_Mode_Enum."All") -> ("error out"=w567:errorcluster, "AD7747 Values"=→"CMin+VCAP":string[][])  [unwired: 7 in]
                  n142 = local write "C1 Min_T0"(w574) -> ()
                  n143 = local write "C3 Min_T0"(w574) -> ()
                  n144 = local write "C2 Min_T0"(w574) -> ()
                  n145 = call "Delay T4.vi"("milliseconds to wait"=u32 100, "error in (no error)"=w567) -> ("error out"=w579:errorcluster)  [unwired: 9 in]
                }
              }
              n146 = case shown="1..3" w498 {
                tunnel: w497 -> [w525 w532]
                tunnel: _ -> [w524 _]
                tunnel: [w515 w532] -> w492
                tunnel: [w513 w535] -> _
                tunnel: [w512 w531] -> _
                tunnel: [w511 w527] -> w493
                tunnel: [w506 "0"] -> _
                tunnel: [w505 w528] -> _
                tunnel: _ -> [w504 w531]
                tunnel: _ -> [w503 w529]
                tunnel: w494 -> [w502 w527]
                tunnel: w491 -> [w501 _]
                frame 1..3 {
                  w518 = u16 0 items=["Voltage", "Current"] ("Source Mode  (0: Voltage)")
                  n147 = Index Array(array=w501, index=w524) -> (element=w508:dbl)
                  n148 = call "Ke2400 Configure Output.vi"("Source Mode  (0: Voltage)"=w518, "error in (no error)"=w525, "Compliance  Level (0.1)"="VSA_IDD(A)", "Output Level (0)"=w508, "VISA resource name"=w502) -> ("error out"=w522:errorcluster, "VISA resource name out"=w520:refnum<visa-resource-name>)  [unwired: 5 in]
                  n149 = call "Ke2400 Enable.vi"("error in (no error)"=w522, "ON/OFF"=TRUE ("Enable Output (T: Enable)"), "VISA resource name"=w520) -> ("error out"=w523:errorcluster, "VISA resource name out"=w511:refnum<visa-resource-name>)  [unwired: 7 in]
                  n150 = Number To Fractional String(number=w508, precision (6)=i16 2) -> (F-format string=w506:string)  [unwired: 2 in]
                  n151 = call "Delay T4.vi"("milliseconds to wait"=u32 50, "error in (no error)"=w523) -> ("error out"=w510:errorcluster)  [unwired: 9 in]
                  n152 = Concatenate Strings(w503, "_Sweeping Voltage on CAP Head... ", w506) -> (w505:string)
                  n153 = call "Ke2000 Reading MilAmp.vi"("error in (no error)"=w510, "VISA resource name"=w504) -> ("error out"=w515:errorcluster, "uA"=w514:string, "VISA resource name out"=w512:refnum<visa-resource-name>)  [unwired: 7 in]
                  "CP_IDD(uA)" <- w514
                  n154 = for {
                    N: 16 -> [_]
                    tunnel: w514 -> [w526]
                    tunnel: [w526] -> w513 mode=indexing
                  }
                }
                frame 0, Default {
                  n155 = Concatenate Strings(w529, "_No Sweeping Voltage on CAP Head... ") -> (w528:string)
                  n156 = for {
                    N: 16 -> [_]
                    tunnel: "0" ("uA") -> [w537]
                    tunnel: [w537] -> w535 mode=indexing
                  }
                }
              }
            }
            frame "Meas_Cap" {
              w588 = FALSE ("Log (T)")
              n157 = call "WS1050 16 DUT AD7747 READ.vi"("Log (T)"=w588, "DUT Mask Mode (All)"=WSVCAP_SHL_I2C_DUT_Mask_Mode_Enum."C1") -> ("error out"=w597:errorcluster, "AD7747 Values"=w599:string[][])  [unwired: 8 in]
              n158 = for {
                tunnel: w599 -> [w621] mode=indexing
                tunnel: [w619] -> w584 mode=indexing
                tunnel: w597 -> [w620]
                tunnel: [w620] -> w596
                n159 = Index Array(array=w621, index=1) -> (element=w619:string)
              }
              n160 = call "WS1050 16 DUT AD7747 READ.vi"("error in"=w596, "Log (T)"=w588, "DUT Mask Mode (All)"=WSVCAP_SHL_I2C_DUT_Mask_Mode_Enum."C2") -> ("error out"=w594:errorcluster, "AD7747 Values"=w593:string[][])  [unwired: 7 in]
              n161 = for {
                tunnel: w593 -> [w617] mode=indexing
                tunnel: [w615] -> w585 mode=indexing
                tunnel: w594 -> [w616]
                tunnel: [w616] -> w592
                n162 = Index Array(array=w617, index=3) -> (element=w615:string)
              }
              n163 = call "WS1050 16 DUT AD7747 READ.vi"("error in"=w592, "Log (T)"=w588, "DUT Mask Mode (All)"=WSVCAP_SHL_I2C_DUT_Mask_Mode_Enum."C3") -> ("error out"=w590:errorcluster, "AD7747 Values"=w589:string[][])  [unwired: 7 in]
              n164 = for {
                tunnel: w589 -> [w613] mode=indexing
                tunnel: [w611] -> w586 mode=indexing
                tunnel: w590 -> [w612]
                tunnel: [w612] -> w587
                n165 = Index Array(array=w613, index=5) -> (element=w611:string)
              }
              n166 = case shown="0" {
                selector: _ -> [_ _]
                tunnel: w587 -> [w603 w610]
                tunnel: [w603 w610] -> _
                tunnel: w586 -> [w600 w607]
                tunnel: w585 -> [w601 w608]
                tunnel: w584 -> [w602 w609]
                tunnel: [w602 w609] -> _
                tunnel: [w601 w608] -> _
                tunnel: [w600 w607] -> _
                tunnel: [w600 w606] -> _
                tunnel: [w601 w605] -> _
                tunnel: [w602 w604] -> _
                frame 0 {
                  "C3 Min_T0" <- w600
                  "C2 Min_T0" <- w601
                  "C1 Min_T0" <- w602
                }
                frame 1, Default {
                  n167 = local read "C3 Min_T0"() -> (w606:string[])
                  n168 = local read "C1 Min_T0"() -> (w604:string[])
                  n169 = local read "C2 Min_T0"() -> (w605:string[])
                }
              }
              n170 = call "WS1050 VSA_Delta C Calculation.vi"() -> ()  [unwired: 9 in, 3 out]
              n171 = call "WS1050 VSA_Delta C Calculation.vi"() -> ()  [unwired: 9 in, 3 out]
              n172 = call "WS1050 VSA_Delta C Calculation.vi"() -> ()  [unwired: 9 in, 3 out]
            }
            frame "Save Data" {
            }
            frame "Plot" {
            }
            frame "Idle...", Default {
            }
          }
        }
        n173 = VISA Write(write buffer="SOUR:FUNC VOLT;VOLT:MODE FIX;RANG 100;LEV 0.0;:SENS:FUNC \"CURR\";CURR:PROT 60E-3;RANG 100E-3;:OUTP ON") -> (VISA resource name out=w257:refnum<visa-resource-name>, error out=w254:errorcluster)  [unwired: 2 in, 1 out]
        n174 = for {
          tunnel: _ -> [w632]
          tunnel: w255 -> [w629] mode=indexing
          shift-right: [w627] -> w252
          shift-left: w254 -> [w633]
          tunnel: [w625] -> w253
          n175 = call "E3631A_Voltage Controller updated.vi"("VISA resource name"=w632, "I_VDD(A)"=0.2, "Channel Controller"=w629, "Voltage 1"=0.0, "Voltage 2"=3.3, "error in (no error)"=w633, "Voltage 3"=-3.3) -> ("VISA resource name out"=w625:refnum<visa-resource-name>, "error out"=w628:errorcluster)  [unwired: 7 in]
          n176 = call "Delay T4.vi"("milliseconds to wait"=u32 100, "error in (no error)"=w628) -> ("error out"=w627:errorcluster)  [unwired: 9 in]
        }
        n177 = flat-sequence {
          tunnel: w252 -> [w634]
          tunnel: [w634] -> w251
          frame #0 {
            n178 = One Button Dialog(message="Test Completed") -> ()  [unwired: 1 in, 1 out]
          }
        }
      }
      frame True {
        w636 = FALSE
      }
    }
    n179 = Wait Until Next ms Multiple(millisecond multiple=u32 100) -> ()  [unwired: 1 out]
    n180 = local write "Abort"(w66) -> ()
    n181 = local write "stop"(w67) -> ()
    n182 = Unbundle By Name(w69) -> ("status"=w84:bool)
    n183 = Compound Arithmetic op=OR(w62, w84, w76) -> (w83:bool)
    "STATUS" <- "Idle...." ("STATUS")
  }
  "Ke2000 Out" <- w33
  "PS1 Out" <- w32
  n184 = call "WS1050_16 DUT VSA Save Data Ver1.3.vi"() -> ()  [unwired: 27 in, 1 out]
  n185 = Get Date/Time In Seconds() -> (seconds since 1Jan1904=w6:timestamp)
  n186 = Get Date/Time String(seconds (now)=w6, want seconds? (F)=TRUE) -> (date string=→"date string":string, time string=→"Previous Time":string)  [unwired: 1 in]
  n187 = flat-sequence {
    tunnel: _ -> [w643]
    tunnel: [w643] -> _
    tunnel: _ -> [w641]
    tunnel: [w642] -> _
    frame #0 {
      n188 = Greater Or Equal?(x=w641, y="Set Stress to\nComplete(Cyc/Min)") -> (x >= y?=w642:bool)
      "Stress \nCompleted(Min)" <- w641
    }
  }
  n189 = local write "Abort"(w17) -> ()
  n190 = local write "stop"(w17) -> ()
  n191 = case shown="True" w30 {
    tunnel: [w645 w647] -> w16
    tunnel: w24 -> [w645 w646]
    frame False {
    }
    frame True {
      n192 = flat-sequence {
        tunnel: w646 -> [w650]
        tunnel: [w649] -> w647
        frame #0 {
          n193 = local write "Online"(FALSE ("Online")) -> ()
          n194 = call "WSVCAP SHL Host TL Close.vi"("error in"=w650) -> ("error out"=w649:errorcluster)  [unwired: 14 in]
        }
      }
    }
  }
  "error out" <- w16
  n195 = VISA Write(VISA resource name=w25, write buffer="SOUR:FUNC VOLT;VOLT:MODE FIX;RANG 100;LEV 0.0;:SENS:FUNC \"CURR\";CURR:PROT 60E-3;RANG 100E-3;:OUTP OFF", error in (no error)=w24) -> (VISA resource name out=→"VISA resource name out":refnum<visa-resource-name>, error out=→"error out 2":errorcluster)  [unwired: 1 out]
